vi "AreaVI.vi"() -> ()   [LabVIEW 2019]
panel:
  out "Result":dbl
  in  "y":dbl
  in  "x":dbl
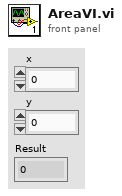
[diagram p1: front panel]
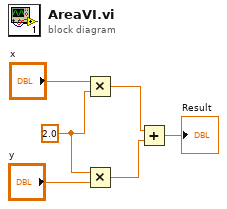
[diagram p0: block diagram]
diagram:
  w5 = 2.0 ("y")
  n1 = Multiply(x="x", y=w5) -> (x*y=w3:dbl)
  n2 = Multiply(x=w5, y="y") -> (x*y=w2:dbl)
  n3 = Add(x=w3, y=w2) -> (x+y=→"Result":dbl)
